vi "Pre Loop Init.vi"() -> ()   [LabVIEW 2019, in "Prueba05.lvclass"]
uses:
  Prueba05.lvclass
  Queues/Private Controls/Queue FGV Action.ctl
  Queues/Private Controls/Prueba5 Estados.ctl
  Queues/Private Controls/Prueba5 Data Cluster.ctl
panel:
  out "error out":errorcluster
  in  "error in (no error)":errorcluster
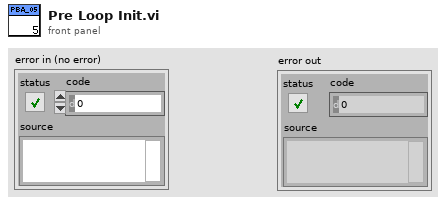
[diagram p1: front panel]
types:
  T1 = typedef "Prueba05.lvclass/Prueba5 Data Cluster.ctl" = cluster{"Estados":T2, "Data":variant}
  T2 = typedef "Prueba05.lvclass/Prueba5 Estados.ctl" = enum16{"inicio", "salir"}
  T3 = typedef "Prueba05.lvclass/Queue FGV Action.ctl" = enum16{"Set", "Get", "Release"}
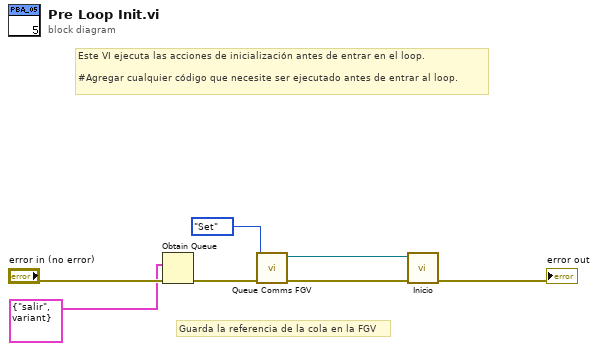
[diagram p0: block diagram]
diagram:
  # "Guarda la referencia de la cola en la FGV"
  # "Este VI ejecuta las acciones de inicialización antes de entrar en el loop.\n\n#Agregar cualquier código que necesite ser ejecutado antes de entrar al loop."
  n1 = Obtain Queue(element data type=T1 {"Estados"=enum."salir", "Data"=variant} ("Element"), error in (no error)="error in (no error)") -> (error out=w6:errorcluster)  [unwired: 3 in, 2 out]
  n2 = call "Queue Comms FGV.vi"("error in (no error)"=w6, "Action"=Queue_FGV_Action."Set") -> ("error out"=w5:errorcluster, "queue out"=w2:refnum<queue>)  [unwired: 8 in]
  n3 = call "Inicio.vi"("error in (no error)"=w5, "Data"=w2) -> ("error out"=→"error out":errorcluster)  [unwired: 9 in]
